vi "AB_API Set Save Settings.vi"(4 "Remove front panel (false)":bool, 6 "Remove block diagram (false)":bool, 8 "error in (no error)":errorcluster, 10 "source item ID":string, 11 "Build in":refnum<class "AB_Build.lvclass">) -> (0 "error out":errorcluster, 3 "Build out":refnum<class "AB_Build.lvclass">)   [LabVIEW 2020]
uses:
  <vilib>/AppBuilder/AB_Classes/Build/AB_Build.lvclass
  <vilib>/AppBuilder/AB_Source_Property_Type.ctl
  <vilib>/AppBuilder/AB_API/common/AB_API Apply Setting Type.ctl
  <vilib>/AppBuilder/AB_Classes/Source/AB_Source.lvclass
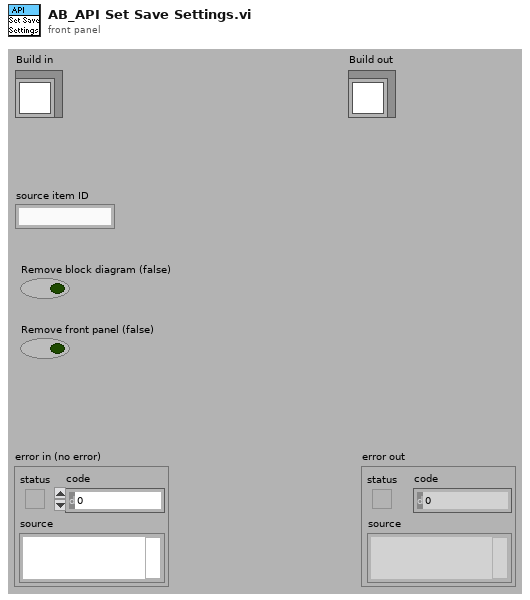
[diagram p1: front panel]
types:
  T1 = typedef "AB_Source_Property_Type.ctl" = enum16{"Remove block diagram", "Remove front panel", "Password", "Window has title bar", "Show menu bar", "Show vertical scroll bar", "Show horizontal scroll bar", "Show toolbar", "Show Abort button", "Show fp when called", "Window behavior", "Allow user to close window", "Window run-time position", "Run when opened", "Allow debugging", "Auto error handling", "Generate guard code", "Use stack variables", "Expression folding", "Integer only", "Inline subVI"}
  T2 = typedef "AB_API Apply Setting Type.ctl" = enum16{"Inclusion", "Destination", "Properties", "Password", "Prefix", "SaveSettings"}
  T3 = typedef "AB_Build.ctl" = cluster{"buildSpecName":string, "buildSpecDescription":string, "destinations":refnum<class "AB_Destination.lvclass">[], "exclusionOption":T4, "defaultLanguage":string, "supportedLanguages":string[], "excludedDirectories":path[], "buildContext":refnum<vi>, "buildObject":T5, "preview":bool, "programatic":bool, "progressBarEvents":T6, "userLog_Path":path, "preActionID":string, "preAction_Path":path, "postActionID":string, "postAction_Path":path, "eng_checkForBrokenVIs?":bool, "eng_verboseLinkerErrors?":bool, "localDest_Path":path, "targetDest_Path":path, "removeVIObject":u16, "cache":refnum<class "PreviewCache.lvclass">, "use cache":bool, "previewCache_ID":string, "buildCache_ID":string, "eng_TempLocalDest_Path":path, "eng_collectDependencies?":bool, "versionInfo":cluster{"buildVersion":cluster{"major":u16, "minor":u16, "patch":u16, "build":u16}, "autoIncrement":bool}, "eng_enableVIChecksums":bool}
  T4 = typedef "AB_Exclusion_Option.ctl" = cluster{"typedefs":bool, "polymorphicVIs":bool, "unusedLibraryItems":bool, "modifyLibraryFile":bool, "edit-timeDependencies":bool, "inlineVIs":bool, "dependent PPLs":bool, "dependent DLLs":bool}
  T5 = typedef "ItemRef.ctl" = u64
  T6 = typedef "provcom_ProgressBar_Events.ctl" = cluster{"newJob":refnum<user-event>, "newItem":refnum<user-event>, "errorMsg":T7, "cancel":refnum<user-event>}
  T7 = typedef "mxLvBuildError.ctl" = refnum<user-event>
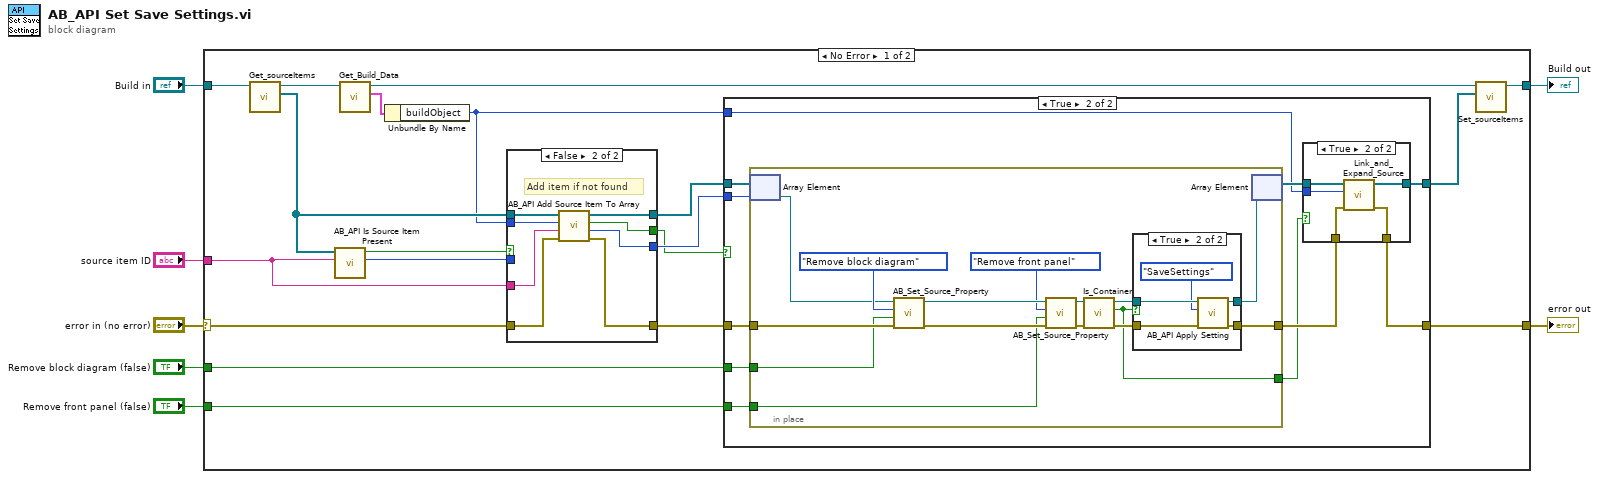
[diagram p0: block diagram]
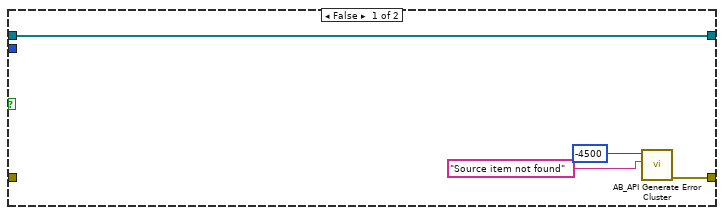
[diagram p3: hidden frame]
diagram:
  n1 = case shown="No Error" "error in (no error)" {
    selector: "error in (no error)" -> [w10 w84]
    tunnel: [w23 w84] -> w6
    tunnel: "Build in" -> [w25 w83]
    tunnel: [w24 w83] -> w4
    tunnel: "source item ID" -> [w12 _]
    tunnel: "Remove block diagram (false)" -> [w22 _]
    tunnel: "Remove front panel (false)" -> [w21 _]
    frame No Error {
      n2 = call <vilib>:"Get_sourceItems.vi"("Class in"=w25) -> ("sourceItems"=w20:refnum<class "AB_Source.lvclass">[], "Class out"=w18:refnum<class "AB_Build.lvclass">)  [unwired: 1 in, 8 out]
      n3 = call <vilib>:"AB_API Is Source Item Present.vi"("item ID"=w12, "source items"=w20) -> ("index"=w13:i32, "source item present?"=w14:bool)  [unwired: 1 in, 7 out]
      n4 = call <vilib>:"Get_Build_Data.vi"("Class in"=w18) -> ("data"=w19:T3, "Class out"=w17:refnum<class "AB_Build.lvclass">)  [unwired: 8 in, 1 out]
      n5 = Unbundle By Name(w19) -> ("buildObject"=w8:T5)
      n6 = case shown="False" w14 {
        selector: w14 -> [w30 _]
        tunnel: [w30 w33] -> w15
        tunnel: w13 -> [w29 _]
        tunnel: [w28 w35] -> w9
        tunnel: w10 -> [w28 w36]
        tunnel: [w29 w34] -> w16
        tunnel: w12 -> [_ w31]
        tunnel: [w27 w37] -> w11
        tunnel: w20 -> [w27 w38]
        tunnel: w8 -> [_ w32]
        frame True {
        }
        frame False {
          # "Add item if not found"
          n7 = call <vilib>:"AB_API Add Source Item To Array.vi"("error in (no error)"=w36, "source item ID"=w31, "buildObject"=w32, "source items in"=w38) -> ("error out"=w35:errorcluster, "index"=w34:i32, "added?"=w33:bool, "source items out"=w37:refnum<class "AB_Source.lvclass">[])  [unwired: 4 in]
        }
      }
      n8 = case shown="True" w15 {
        tunnel: w9 -> [_ w53]
        tunnel: [w40 w45] -> w23
        tunnel: w11 -> [w39 w52]
        tunnel: w16 -> [_ w51]
        tunnel: [w39 w47] -> w26
        tunnel: w21 -> [_ w50]
        tunnel: w22 -> [_ w49]
        tunnel: w8 -> [_ w44]
        frame False {
          n9 = call <vilib>:"AB_API Generate Error Cluster.vi"("Additional Message"="Source item not found", "Code"=-4500) -> ("error out"=w40:errorcluster)  [unwired: 2 in, 7 out]
        }
        frame True {
          n10 = in-place {
            in-place-border: w53 -> [w70]
            in-place-border: [w62] -> w46
            in-place-border: w49 -> [w69]
            in-place-border: w50 -> [w68]
            in-place-border: [w61] -> w43
            n11 = in-place-array #1(w52, w51) -> (w71:refnum<class "AB_Source.lvclass">)
            n12 = call <vilib>:"AB_Set_Source_Property.vi"("error in (no error)"=w70, "property value"=w69, "property name"=AB_Source_Property_Type."Remove block diagram", "Source in"=w71) -> ("error out"=w74:errorcluster, "Source out"=w75:refnum<class "AB_Source.lvclass">)  [unwired: 6 out]
            n13 = call <vilib>:"AB_Set_Source_Property.vi"("error in (no error)"=w74, "property value"=w68, "property name"=AB_Source_Property_Type."Remove front panel", "Source in"=w75) -> ("error out"=w63:errorcluster, "Source out"=w65:refnum<class "AB_Source.lvclass">)  [unwired: 6 out]
            n14 = call-dynamic "Is_Container.vi"("error in (no error)"=w63, "AB_Source in"=w65) -> ("error out"=w66:errorcluster, "container"=w61:bool, "AB_Source out"=w67:refnum<class "AB_Source.lvclass">)  [unwired: 7 in]
            n15 = case shown="True" w61 {
              tunnel: [w77 w82] -> w64
              tunnel: [w76 w81] -> w62
              tunnel: w67 -> [w77 w80]
              tunnel: w66 -> [w76 w79]
              frame False {
              }
              frame True {
                n16 = call <vilib>:"AB_API Apply Setting.vi"("error in (no error)"=w79, "Settings"=AB_API_Apply_Setting_Type."SaveSettings", "Source in"=w80) -> ("error out"=w81:errorcluster, "Source out"=w82:refnum<class "AB_Source.lvclass">)  [unwired: 7 in]
              }
            }
            n17 = in-place-array #1(w64) -> (w48:refnum<class "AB_Source.lvclass">[])  [unwired: 1 out]
          }
          n18 = case shown="True" w43 {
            tunnel: w48 -> [w55 w60]
            tunnel: [w55 w59] -> w47
            tunnel: w44 -> [_ w58]
            tunnel: w46 -> [w54 w57]
            tunnel: [w54 w56] -> w45
            frame False {
            }
            frame True {
              n19 = call <vilib>:"Link_and_Expand_Source.vi"("error in (no error)"=w57, "Object"=w58, "AB_Source in"=w60) -> ("error out"=w56:errorcluster, "AB_Source out"=w59:refnum<class "AB_Source.lvclass">[])  [unwired: 7 in]
            }
          }
        }
      }
      n20 = call <vilib>:"Set_sourceItems.vi"("sourceItems"=w26, "Class in"=w17) -> ("Class out"=w24:refnum<class "AB_Build.lvclass">)  [unwired: 1 in, 8 out]
    }
    frame Error {
    }
  }
  "error out" <- w6
  "Build out" <- w4
